vi "HDI Start Position Verify.vi"() -> ()   [LabVIEW 2011]
uses:
  Shared Components/Gantry Class/Gantry Class.lvclass
  Shared Components/WorkTable Class/WorkTable Class.lvclass
  Shared Components/Vec3d Class/Vec3d Class.lvclass
panel:
  in  "Quit":bool
  out "Current fiducial":string
  out "error out":errorcluster
  out "preview":T1(plugin-control)
  out "Current Position":cluster{"X":dbl, "Y":dbl, "Z":dbl}
  in  "Slot Number":u32
  in  "Next":bool
  in  "Config Folder":path=path "C:/Users/Husker/Desktop/gantry/Config"
  # "Set this to the appropriate slot number *before* running"
  # "Press this button to go to \nnext fiducial"
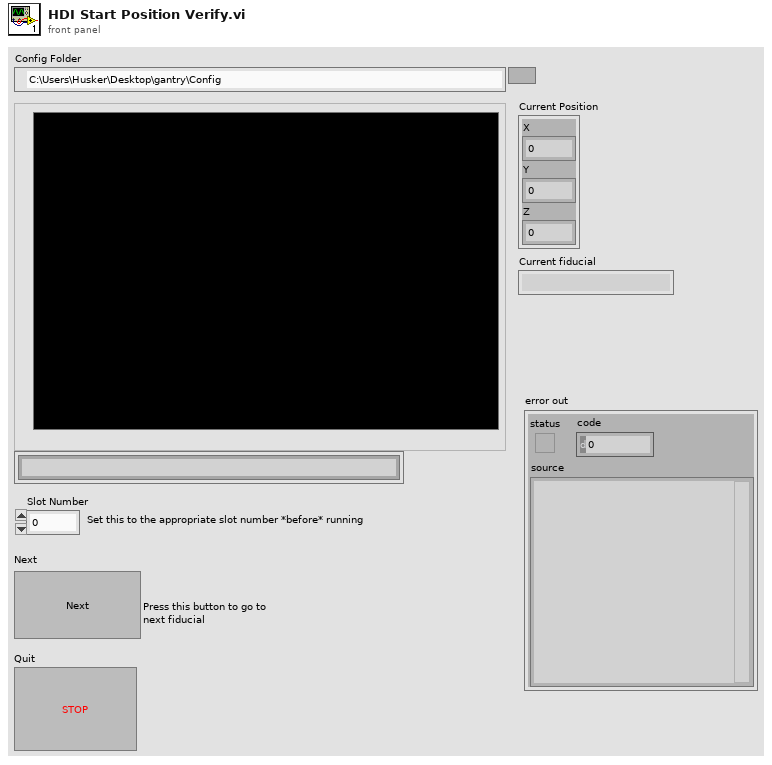
[diagram p1: front panel]
types:
  T1 = typedef "IMAQ Image.ctl" = refnum<image>
  T2 = typedef "Image Type" = u32
  T3 = typedef "Worktable_HDI Slot.ctl" = cluster{"HDI Assembly State":enum16{"Empty", "Populated"}, "HDI Type":enum16{"HDI", "Polyimide"}, "Vacuum Channel":u32, "Location/Orientation":T4}
  T4 = typedef "Position_Orientation.ctl" = cluster{"Center":refnum<class "Vec3d Class.lvclass">, "Orientation":refnum<class "Orient3d Class.lvclass">}
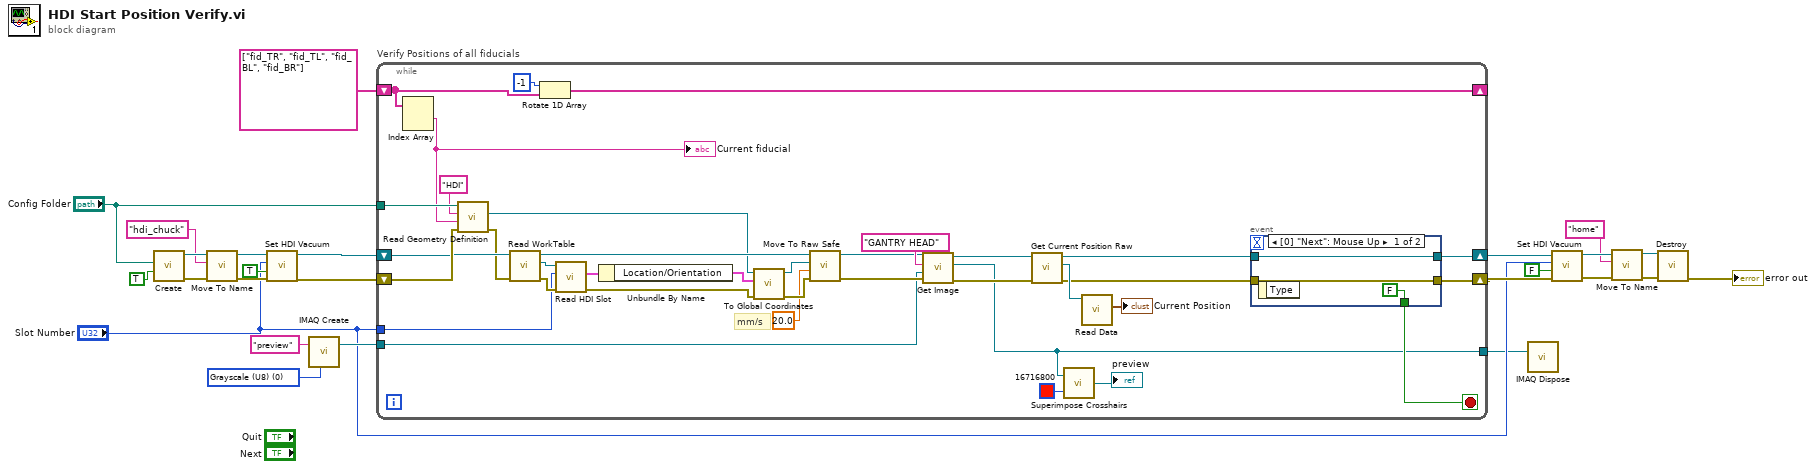
[diagram p0: block diagram]
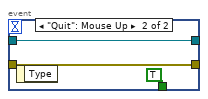
[diagram p2: hidden frame]
diagram:
  w21 = T2 0 items=["Grayscale (U8)", "Grayscale (I16)", "Grayscale (SGL)", "Complex (CSG)", "RGB (U32)", "HSL (U32)", "RGB (U64)", "Grayscale (U16)"] ("Image Type")
  n1 = call "Create.vi"("HOME?"=TRUE, "Config Folder"="Config Folder") -> ("error out"=w18:errorcluster, "Gantry out"=w16:refnum<class "Gantry Class.lvclass">)  [unwired: 8 in]
  n2 = call-dynamic "Move To Name.vi"("error in"=w18, "Destination Name"="hdi_chuck", "Gantry in"=w16) -> ("error out"=w17:errorcluster, "Gantry out"=w15:refnum<class "Gantry Class.lvclass">)  [unwired: 7 in]
  n3 = call-dynamic "Set HDI Vacuum.vi"("error in"=w17, "On/Off"=TRUE, "Slot Number"="Slot Number", "Gantry in"=w15) -> ("error out"=w11:errorcluster, "Gantry out"=w12:refnum<class "Gantry Class.lvclass">)  [unwired: 6 in]
  n4 = call "IMAQ Create"("Image Name"="preview", "Image Type"=w21) -> ("New Image"=w19:T1)  [unwired: 3 in, 1 out]
  n5 = while "Verify Positions of all fiducials" {
    tunnel: "Config Folder" -> [w61]
    shift-right: [w34] -> w10
    shift-left: w12 -> [w48]
    shift-right: [w32] -> w9
    shift-left: w11 -> [w59]
    tunnel: w19 -> [w27]
    shift-right: [w58] -> _
    shift-left: string[] ["fid_TR", "fid_TL", "fid_BL", "fid_BR"] -> [w57]
    tunnel: "Slot Number" -> [w44]
    tunnel: [w26] -> w1
    stop <- w29 stop-if-true
    # "mm/s"
    n6 = Index Array(array=w57) -> (element #1=w30:string)  [unwired: 2 in, 1 out]
    "Current fiducial" <- w30
    n7 = call "Read Geometry Definition.vi"("error in"=w59, "Feature"=w30, "Part"="HDI", "Config Location"=w61) -> ("error out"=w47:errorcluster, "Feature Coordinates"=w36:refnum<class "Vec3d Class.lvclass">)  [unwired: 6 in]
    n8 = call-dynamic "Read WorkTable.vi"("error in"=w47, "Gantry Class in"=w48) -> ("error out"=w46:errorcluster, "WorkTable Class.lvclass"=w45:refnum<class "WorkTable Class.lvclass">, "Gantry Class out"=w40:refnum<class "Gantry Class.lvclass">)  [unwired: 7 in]
    n9 = Rotate 1D Array(1:w57, 2:-1 ("n")) -> (0:w58:string[])
    n10 = call-dynamic "Read HDI Slot.vi"("error in"=w46, "HDI Slot Number"=w44, "WorkTable in"=w45) -> ("error out"=w41:errorcluster, "HDI Slot"=w43:T3)  [unwired: 6 in, 1 out]
    n11 = Unbundle By Name(w43) -> ("Location/Orientation"=w42:T4)
    n12 = call "To Global Coordinates.vi"("error in"=w41, "Center/Orientation"=w42, "Local Coordinates"=w36) -> ("error out"=w38:errorcluster, "Global Coordinates"=w35:refnum<class "Vec3d Class.lvclass">)  [unwired: 7 in]
    n13 = call-dynamic "Move To Raw Safe.vi"("error in"=w38, "Speed"=20.0, "Destination"=w35, "Gantry in"=w40) -> ("error out"=w37:errorcluster, "Gantry out"=w39:refnum<class "Gantry Class.lvclass">)  [unwired: 6 in]
    n14 = call-dynamic "Get Image.vi"("error in"=w37, "Image In"=w27, "Camera Name"="GANTRY HEAD", "Gantry in"=w39) -> ("error out"=w53:errorcluster, "Image Out"=w26:T1, "Gantry out"=w54:refnum<class "Gantry Class.lvclass">)  [unwired: 4 in, 1 out]
    n15 = call-dynamic "Get Current Position Raw.vi"("error in (no error)"=w53, "Gantry Class in"=w54) -> ("error out"=w31:errorcluster, "Vec3d Class out"=w52:refnum<class "Vec3d Class.lvclass">, "Gantry Class out"=w33:refnum<class "Gantry Class.lvclass">)  [unwired: 7 in]
    n16 = call "Superimpose Crosshairs.vi"("Grid Line Color"=u32 16716800, "Refnum in"=w26) -> ("Refnum out"=→"preview":T1)
    n17 = call-dynamic "Read Data.vi"("Vec3d Class in"=w52) -> ("Data"=→"Current Position":cluster{"X":dbl, "Y":dbl, "Z":dbl})  [unwired: 8 in, 2 out]
    n18 = event shown="[0] \"Next\": Mouse Up" {
      selector: _ -> [_ _]
      dyn-events: _ -> [_ _]
      timeout: _ -> [_ _]
      tunnel: [w64 w67] -> w34
      tunnel: w33 -> [w64 w67]
      tunnel: [w63 w66] -> w32
      tunnel: w31 -> [w63 w66]
      tunnel: [FALSE TRUE] -> w29
      event "Next": Mouse Up {
        n19 = event-data() -> ()  [unwired: 1 in, 1 out]
      }
      event "Quit": Mouse Up {
        n20 = event-data() -> ()  [unwired: 1 in, 1 out]
      }
    }
  }
  n21 = call "IMAQ Dispose"("Image"=w1) -> ()  [unwired: 5 in, 1 out]
  n22 = call-dynamic "Set HDI Vacuum.vi"("error in"=w9, "On/Off"=FALSE, "Slot Number"="Slot Number", "Gantry in"=w10) -> ("error out"=w4:errorcluster, "Gantry out"=w6:refnum<class "Gantry Class.lvclass">)  [unwired: 6 in]
  n23 = call-dynamic "Move To Name.vi"("error in"=w4, "Destination Name"="home", "Gantry in"=w6) -> ("error out"=w3:errorcluster, "Gantry out"=w5:refnum<class "Gantry Class.lvclass">)  [unwired: 7 in]
  n24 = call "Destroy.vi"("error in"=w3, "Gantry Class in"=w5) -> ("error out"=→"error out":errorcluster)  [unwired: 9 in]
